vi "Register for Remote Messages.vi"(7 "Force (F)":bool, 8 "error in (no error)":errorcluster, 10 "Messages":T1[](array[typedef]), 11 "Module in":refnum<class "Module.lvclass">) -> (0 "error out":errorcluster, 3 "Module out":refnum<class "Module.lvclass">)   [LabVIEW 2020, in "Volatus.lvlib" / "Module.lvclass"]
uses:
  Module.lvclass
  Message Registration.ctl
  Module.lvclass/Module.ctl
  Messages Registration.ctl
  MessageQ/MessageQ.lvclass
  Remote Messaging Identity/Remote Messaging Identity.lvclass
  C:/dev/lv20CE/relink/lv-volatus/Volatus/Identity/Identity.lvclass
  Event Level.ctl
  MessageQ/MessageQ.lvclass/MessageQ.ctl
  Volatus.lvlib
  VolatusAPI/VolatusAPI.lvclass
  C:/dev/lv20CE/relink/lv-volatus/Volatus/Remote Messaging Identity/Remote Messaging Identity.lvclass
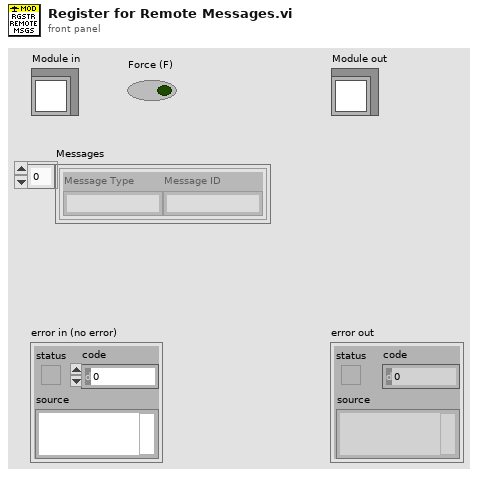
[diagram p1: front panel]
types:
  T1 = typedef "Volatus.lvlib/Message Registration.ctl" = cluster{"Message Type":string, "Message ID":string}
  T2 = typedef "Volatus.lvlib/Messages Registration.ctl" = cluster{"MessageQ":refnum<class "MessageQ.lvclass">, "Messages":T1[]}
  T3 = typedef "Volatus.lvlib/Event Level.ctl" = enum16{"Debug", "Info", "Warning", "Error"}
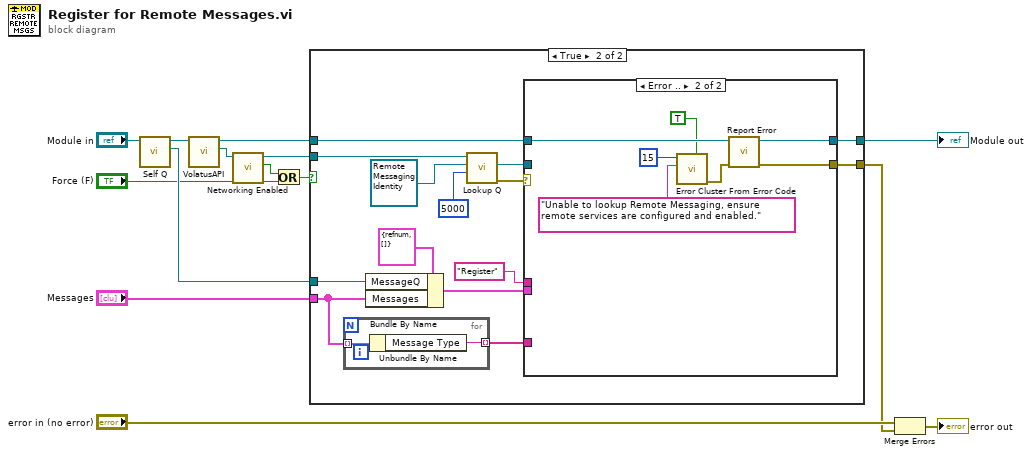
[diagram p0: block diagram]
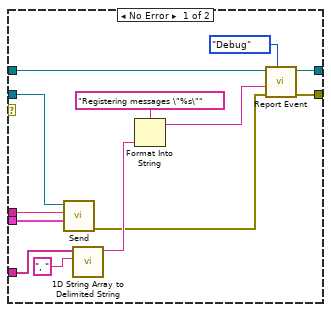
[diagram p3: hidden frame]
diagram:
  n1 = call "Self Q.vi"("Module in"="Module in") -> ("Self Q"=w11:refnum<class "MessageQ.lvclass">, "Module out"=w12:refnum<class "Module.lvclass">)  [unwired: 9 in]
  n2 = call "VolatusAPI.vi"("Module in"=w12) -> ("VolatusAPI"=w10:refnum<class "VolatusAPI.lvclass">, "Module out"=w9:refnum<class "Module.lvclass">)  [unwired: 9 in]
  n3 = call "Networking Enabled.vi"("VolatusAPI in"=w10) -> ("Networking Enabled"=w3:bool, "VolatusAPI out"=w4:refnum<class "VolatusAPI.lvclass">)  [unwired: 9 in]
  n4 = Or(x=w3, y="Force (F)") -> (x .or. y?=w2:bool)
  n5 = case shown="True" w2 {
    tunnel: w11 -> [_ w27]
    tunnel: w4 -> [_ w26]
    tunnel: w9 -> [w15 w21]
    tunnel: [_ w20] -> w7
    tunnel: [w15 w19] -> w6
    tunnel: "Messages" -> [_ w18]
    frame False {
    }
    frame True {
      n6 = for {
        tunnel: w18 -> [w51] mode=indexing
        tunnel: [w50] -> w17 mode=indexing
        n7 = Unbundle By Name(w51) -> ("Message Type"=w50:string)
      }
      n8 = Bundle By Name(cluster=T2 {"MessageQ"=refnum, "Messages"=[]} ("Messages Registration"), "MessageQ"=w27, "Messages"=w18) -> (w24:T2)
      n9 = call "Lookup Q.vi"("Timeout ms (0)"=5000, "Identity"=refnum<class "Remote Messaging Identity.lvclass"> refnum ("Volatus:Remote Messaging Identity.lvclass"), "VolatusAPI in"=w26) -> ("error out"=w29:errorcluster, "MessageQ"=w23:refnum<class "MessageQ.lvclass">)  [unwired: 6 in, 1 out]
      n10 = case shown="Error .." w29 {
        tunnel: w24 -> [w42 _]
        tunnel: w23 -> [w41 _]
        tunnel: "Register" ("ID") -> [w40 _]
        tunnel: w21 -> [w39 w47]
        tunnel: [w30 w45] -> w20
        tunnel: [w38 w44] -> w19
        tunnel: w17 -> [w36 _]
        frame No Error {
          n11 = call "Send.vi"("Data"=w42, "ID"=w40, "MessageQ in"=w41) -> ("error out"=w31:errorcluster)  [unwired: 7 in, 1 out]
          n12 = call <vilib>:"1D String Array to Delimited String.vi"("delimiter"=", ", "string array"=w36) -> ("delimited string"=w33:string)  [unwired: 9 in]
          n13 = Format Into String(format string="Registering messages \"%s\"", w33) -> (resulting string=w32:string)  [unwired: 2 in, 1 out]
          n14 = call "Report Event.vi"("Level (Info)"=Event_Level."Debug", "error in (no error)"=w31, "Message"=w32, "Module in"=w39) -> ("error out"=w30:errorcluster, "Module out"=w38:refnum<class "Module.lvclass">)  [unwired: 6 in]
        }
        frame Error {
          n15 = call <vilib>:"Error Cluster From Error Code.vi"("is warning? (False)"=TRUE, "error message (\"\")"="Unable to lookup Remote Messaging, ensure remote services are configured and enabled." ("error message (\"\")"), "error code (0)"=15) -> ("error out"=w46:errorcluster)  [unwired: 6 in]
          n16 = call "Report Error.vi"("error in (no error)"=w46, "Module in"=w47) -> ("error out"=w45:errorcluster, "Module out"=w44:refnum<class "Module.lvclass">)  [unwired: 8 in]
        }
      }
    }
  }
  "Module out" <- w6
  n17 = Merge Errors("error in (no error)", w7) -> (→"error out":errorcluster)
